vi "Teleop.vi"(10 "Match Info":T1={"Autonomous Elapsed Seconds"=0.0, "TeleOp Elapsed Seconds"=59.323, "Disabled Elapsed Seconds"=2.887, "Visited Autonomous"=FALSE, "Visited TeleOp"=TRUE, "Visited Disabled"=TRUE, "Autonomous Settings"={"Autonomous Style"=enum."Independent", "VI Refnum"=refnum}}, 11 "Call Context":T2=enum."Stop") -> ()   [LabVIEW 2018]
doc: "This VI is called for each enabled TeleOp packet received from the DS. It is typically used to read from joysticks and other inputs and update I/O or setpoints for timed control loops. It should complete and return within 20 milliseconds or risk missing DS packets."
uses:
  <vilib>/Rock Robotics/WPI/DriverStation/WPI_DriverStationDerivedRobotMode.ctl
  <vilib>/Rock Robotics/WPI/DriverStation/WPI_DriverStationMatch Info.ctl
  Typedef/XBox Axis.ctl
  Typedef/XBox Buttons.ctl
  <vilib>/Rock Robotics/WPI/ThirdParty/REV Robotics/SPARK MAX/Typedef/Spark MAX Idle Mode.ctl
  <vilib>/Rock Robotics/WPI/Solenoid/WPI_SolenoidValue.ctl
  <vilib>/Rock Robotics/WPI/Utilities/WPI_GetSetVariantRefNum.vi
  <vilib>/Rock Robotics/Network Tables/NT Write Boolean Array.vi
  <vilib>/Rock Robotics/Network Tables/NT Write Numeric Array.vi
  <vilib>/Rock Robotics/Network Tables/NT Read Number.vi
  <vilib>/Rock Robotics/Network Tables/NT Write Number.vi
  <vilib>/Rock Robotics/WPI/Solenoid/WPI_SolenoidSetEnum.vi
  Beak/Implementation/Beak Published Globals.vi
  Wrist/Implementation/Wrist Published Globals.vi
panel:
  in  "Max Acceleration":dbl=800.0
  in  "Max Velocity":dbl=400.0
  in  "Arm angle from 'Y'":dbl=86.0 format="%#_13g"
  in  "Joystick Deadband":dbl=0.07 format="%#_13g"
  in  "Throttle Sensitivity":dbl(slide)=0.7142857142857142 scale=0.0..1.0
  in  "Elevator Speed":dbl=1.5 format="%#_13g"
  in  "QuesoTurn Sensitivty":dbl=0.7
  in  "Cheesy Sensitivity":dbl(slide)=0.5864661654135338 scale=0.0..1.0
  in  "Arcade to Queso":bool=TRUE
  # "<-- This is not motor speed!"
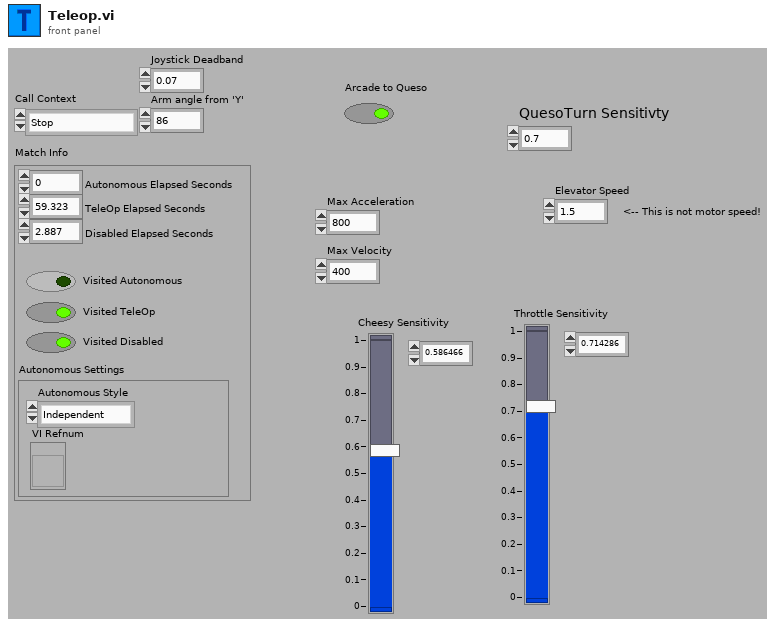
[diagram p1: front panel]
types:
  T1 = typedef "WPI_DriverStationMatch Info.ctl" = cluster{"Autonomous Elapsed Seconds":dbl, "TeleOp Elapsed Seconds":dbl, "Disabled Elapsed Seconds":dbl, "Visited Autonomous":bool, "Visited TeleOp":bool, "Visited Disabled":bool, "Autonomous Settings":cluster{"Autonomous Style":enum16{"Iterative", "Independent"}, "VI Refnum":refnum<vi>}}
  T2 = typedef "WPI_DriverStationDerivedRobotMode.ctl" = enum16{"Init", "Execute", "Stop"}
  T3 = typedef "XBox Buttons.ctl" = enum16{"A", "B", "X", "Y", "Left Bumper", "Right Bumper", "Back", "Start", "Left Joystick", "Right Joystick"}
  T4 = typedef "XBox Axis.ctl" = enum16{"Left X", "Left Y", "Left Trigger", "Right Trigger", "Right X", "Right Y"}
  T5 = typedef "WPI_JoystickDevRef.ctl" = cluster{"Device":T6}
  T6 = typedef "WPI_JoystickDeviceEnum.ctl" = enum16{"USB 0", "USB 1", "USB 2", "USB 3", "USB 4", "USB 5"}
  T7 = typedef "Spark MAX Idle Mode.ctl" = enum16{"Coast", "Brake"}
  T8 = typedef "SPARKMAX6Motor.ctl" = cluster{"FrontLeftMaster":T9, "FrontLeftSlave1":T9, "FrontLeftSlave2":T9, "FrontRightMaster":T9, "FrontRightSlave1":T9, "FrontRightSlave2":T9}
  T9 = typedef "WPI_MotorControlDeviceRef.ctl" = cluster{"DeviceStatus":errorcluster, "Type":T10, "PWM":cluster{"PWM Channel":T11, "DeadBand":T12}, "CAN":cluster{"Device Number":u8, "SetOutput VI Ref":variant, "GetOutput VI Ref":variant, "Enable VI Ref":variant, "Disable VI Ref":variant, "Data":variant}, "Invert":bool, "DIO PWM":cluster{"PWM \"Enable\" Channel":T11, "DIOChannel":T13, "PWM Rate":dbl}}
  T10 = typedef "WPI_MotorControlType.ctl" = enum16{"PWM", "CAN", "DIO PWM"}
  T11 = typedef "FPGA_DIOPWMChannel.ctl" = enum8{"PWM 0", "PWM 1", "PWM 2", "PWM 3", "PWM 4", "PWM 5", "PWM 6", "PWM 7", "PWM 8", "PWM 9", "PWM MXP 0", "PWM MXP 1", "PWM MXP 2", "PWM MXP 3", "PWM MXP 4", "PWM MXP 5", "PWM MXP 6", "PWM MXP 7", "PWM MXP 8", "PWM MXP 9", "Invalid"}
  T12 = typedef "WPI_PWMDeadband.ctl" = cluster{"Name":string, "maxPositivePwm":i32, "minPositivePwm":i32, "centerPwm":i32, "maxNegativePwm":i32, "minNegativePwm":i32, "angularRange":u16}
  T13 = typedef "FPGA_DIOChannel.ctl" = enum8{"DIO 0", "DIO 1", "DIO 2", "DIO 3", "DIO 4", "DIO 5", "DIO 6", "DIO 7", "DIO 8", "DIO 9", "DIO MXP 0", "DIO MXP 1", "DIO MXP 2", "DIO MXP 3", "DIO MXP 4", "DIO MXP 5", "DIO MXP 6", "DIO MXP 7", "DIO MXP 8", "DIO MXP 9", "DIO MXP 10", "DIO MXP 11", "DIO MXP 12", "DIO MXP 13", "DIO MXP 14", "DIO MXP 15", "SPI Port CS1", "SPI Port CS2", "SPI Port CS3", "SPI Port MISO", "SPI Port MOSI", "Invalid"}
  T14 = typedef "WPI_SolenoidValue.ctl" = enum16{"Off", "On", "Forward", "Reverse"}
  T15 = typedef "WPI_SolenoidDevRef.ctl" = cluster{"DevStatus":errorcluster, "Pneumatics Control Module":u8, "Forward Solenoid Channel":T16, "Reverse Solenoid Channel":T16}
  T16 = typedef "WPI_SolenoidChannel.ctl" = enum8{"Solenoid 0", "Solenoid 1", "Solenoid 2", "Solenoid 3", "Solenoid 4", "Solenoid 5", "Solenoid 6", "Solenoid 7", "Invalid"}
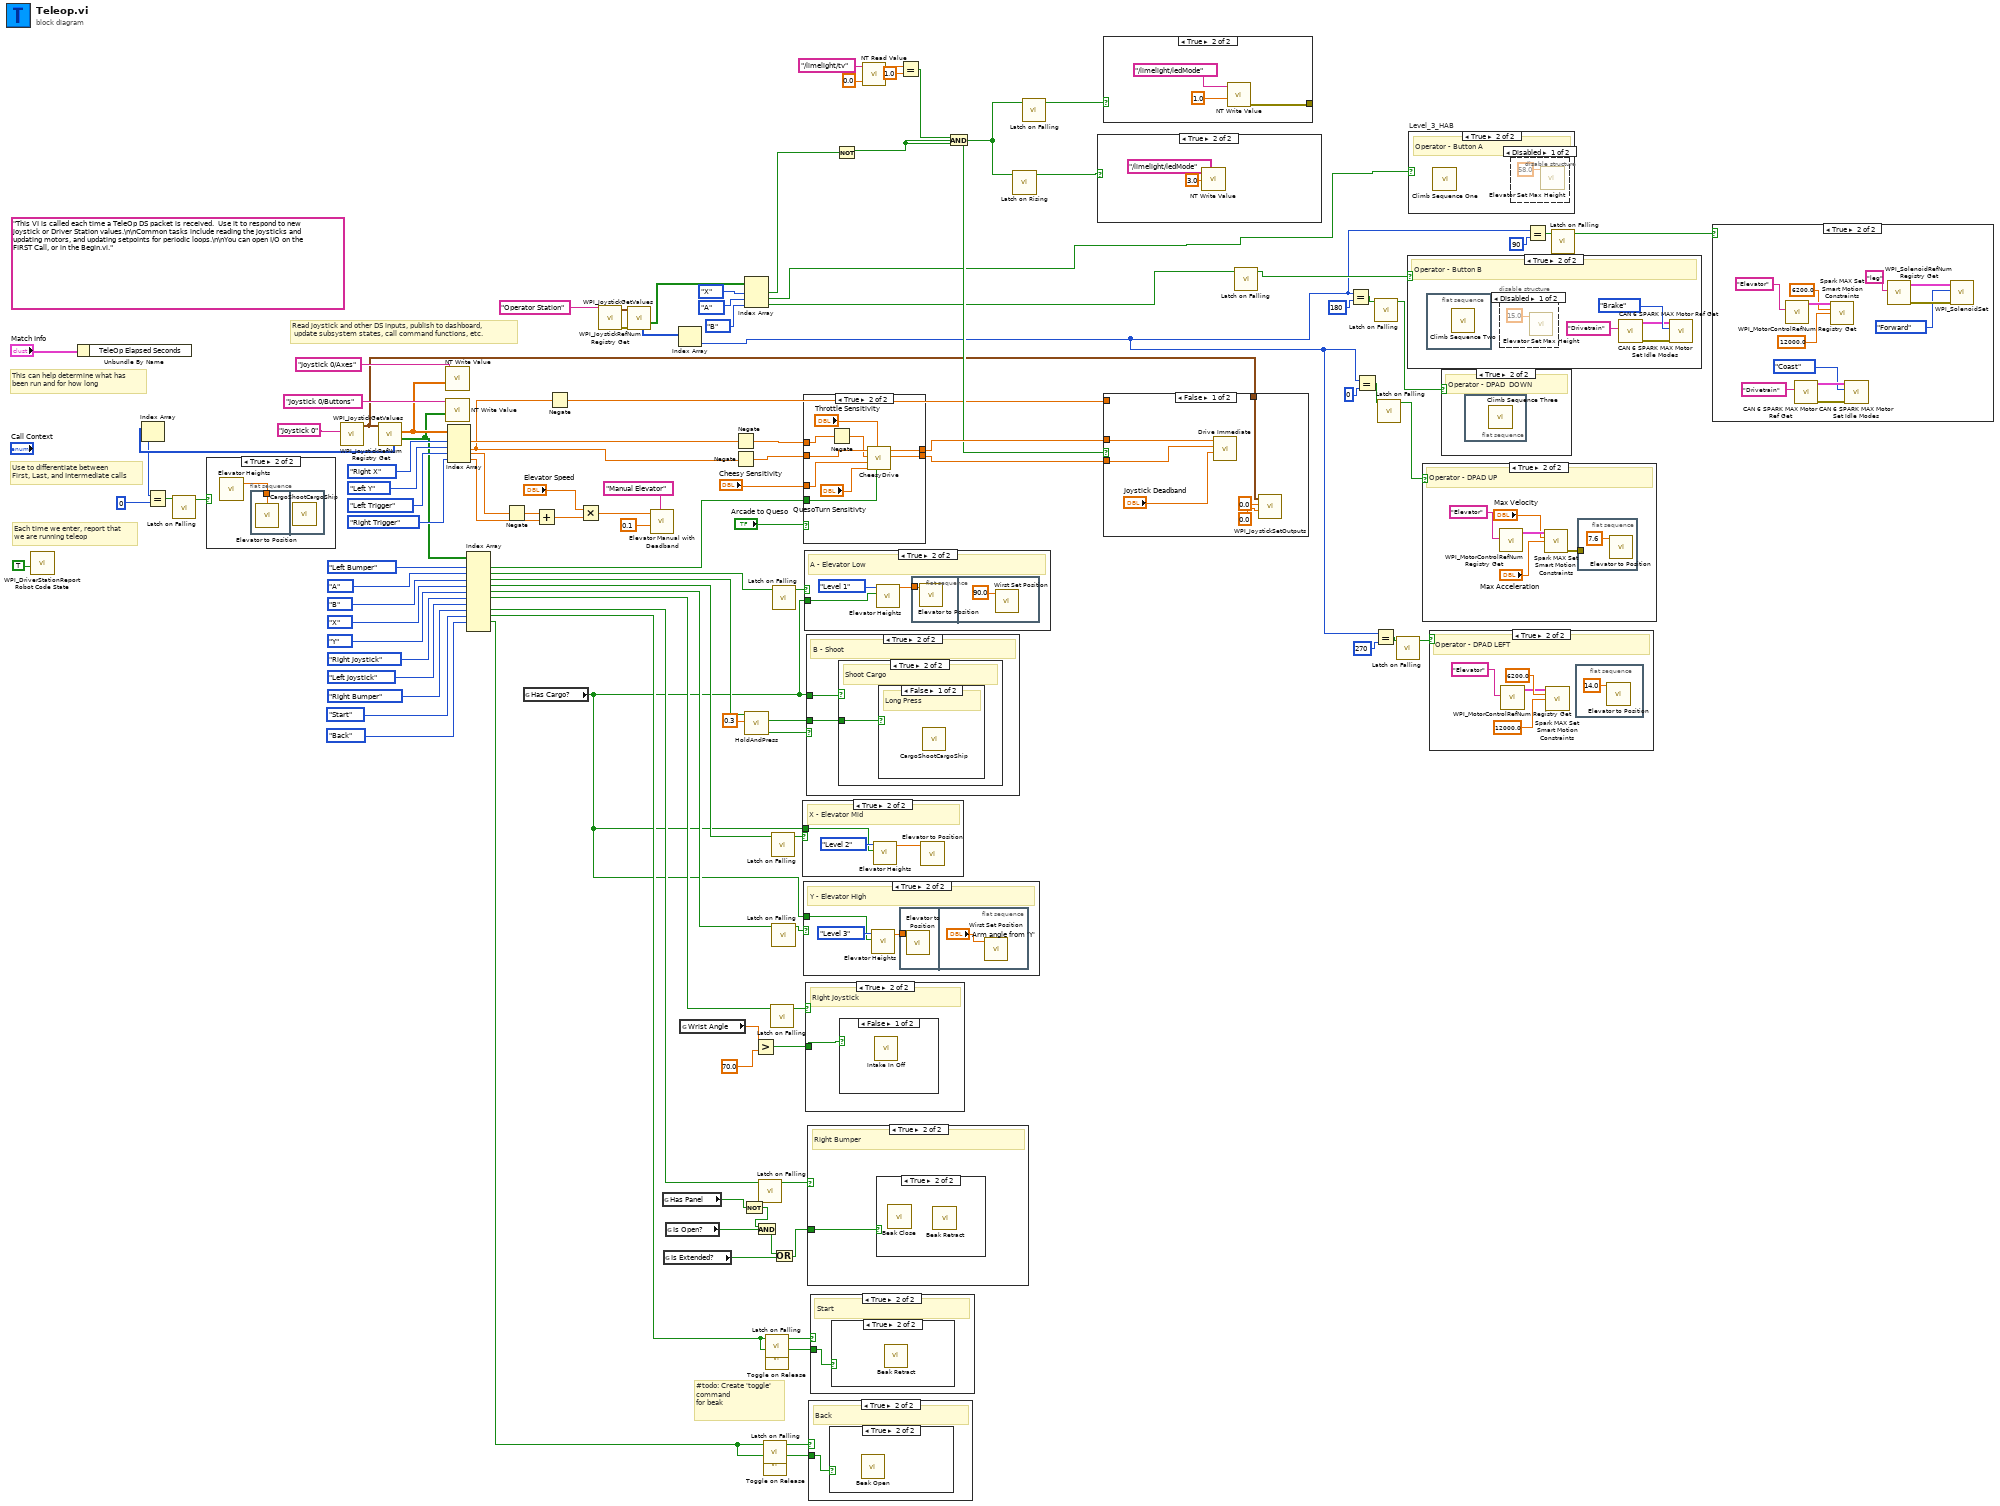
[diagram p0: block diagram]
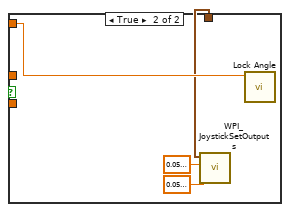
[diagram p13: hidden frame]
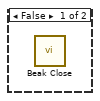
[diagram p16: hidden frame]
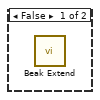
[diagram p18: hidden frame]
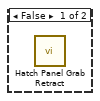
[diagram p20: hidden frame]
diagram:
  (unwired) "This VI is called each time a TeleOp DS packet is received.  Use it to respond to new joystick or Driver Station values.\n\nCommon tasks include reading the joysticks and updating motors, and updating setpoints for periodic loops.\n\nYou can open I/O on the FIRST Call, or in the Begin.vi."
  # "#todo: Create 'toggle' command\nfor beak"
  # "Read joystick and other DS inputs, publish to dashboard,\n update subsystem states, call command functions, etc."
  # "Each time we enter, report that\nwe are running teleop"
  # "Use to differentiate between\nFirst, Last, and Intermediate calls"
  # "This can help determine what has\nbeen run and for how long"
  n1 = call <vilib>:"WPI_DriverStationReport Robot Code State.vi"("TeleOp"=TRUE ("Autonomous")) -> ()  [unwired: 10 in, 1 out]
  n2 = Unbundle By Name("Match Info") -> ()  [unwired: 1 out]
  n3 = call <vilib>:"WPI_JoystickRefNum Registry Get.vi"("refnum name"="Joystick 0") -> ("JoystickDevRef"=w30:T5)  [unwired: 1 in, 9 out]
  n4 = call <vilib>:"WPI_JoystickGetValues.vi"("JoystickDevRef"=w30) -> ("Buttons"=w84:bool[], "Axes"=w105:dbl[], "POVs"=w19:i16[])  [unwired: 6 in, 2 out]
  n5 = Index Array(array=w19) -> (element=w18:i16)  [unwired: 1 in]
  n6 = Equal?(x=w18, y=0) -> (x = y?=w17:bool)
  n7 = call "Latch on Falling.vi"("Boolean in"=w17) -> ("Boolean out"=w16:bool)  [unwired: 4 in]
  n8 = case shown="True" w16 {
    frame False {
    }
    frame True {
      n9 = call "Elevator Heights.vi"() -> ("Cargo Ship Height"=w110:dbl)  [unwired: 10 in, 1 out]
      n10 = flat-sequence {
        tunnel: w110 -> [w111]
        frame #0 {
          n11 = call "Elevator to Position.vi"("Elevator Height"=w111) -> ()  [unwired: 10 in, 1 out]
        }
        frame #1 {
          n12 = call "CargoShootCargoShip.vi"() -> ()  [unwired: 11 in, 1 out]
        }
      }
    }
  }
  n13 = call-poly <vilib>:"NT Write Value.vi"("Numeric Array"=w105, "Name"="Joystick 0/Axes") -> ()  [unwired: 9 in, 1 out]
  n14 = call-poly <vilib>:"NT Write Value.vi"("Boolean Array"=w84, "Name"="Joystick 0/Buttons") -> ()  [unwired: 9 in, 1 out]
  n15 = Index Array(array=w105, index #1=XBox_Axis."Right X" ("Enum"), index #2=XBox_Axis."Left Y" ("Enum"), index #3=XBox_Axis."Left Trigger" ("Enum"), index #4=XBox_Axis."Right Trigger" ("Enum")) -> (element #1=w101:dbl, element #2=w29:dbl, element #3=w89:dbl, element #4=w88:dbl)
  n16 = Index Array(array=w84, index #1=XBox_Buttons."Left Bumper" ("Enum"), index #2=XBox_Buttons."A" ("Enum"), index #3=XBox_Buttons."B" ("Enum"), index #4=XBox_Buttons."X" ("Enum"), index #5=XBox_Buttons."Y" ("Enum"), index #6=XBox_Buttons."Right Joystick" ("Enum"), index #7=XBox_Buttons."Left Joystick" ("Enum"), index #8=XBox_Buttons."Right Bumper" ("Enum"), index #9=XBox_Buttons."Start" ("Enum"), index #10=XBox_Buttons."Back" ("Enum")) -> (element #1=w77:bool, element #2=w76:bool, element #3=w59:bool, element #4=w73:bool, element #5=w72:bool, element #6=w60:bool, element #8=w68:bool, element #9=w64:bool, element #10=w61:bool)  [unwired: 1 in, 2 out]
  n17 = Negate(x=w89) -> (-x=w86:dbl)
  n18 = global read "Wrist Published Globals.vi" "Has Cargo?"() -> (w49:bool)
  n19 = Add(x=w86, y=w88) -> (x+y=w87:dbl)
  n20 = Negate(x=w29) -> (-x=w28:dbl)
  n21 = Multiply(x="Elevator Speed", y=w87) -> (x*y=w80:dbl)
  n22 = call <vilib>:"WPI_JoystickRefNum Registry Get.vi"("refnum name"="Operator Station") -> ("error out"=w44:errorcluster, "JoystickDevRef"=w43:T5)  [unwired: 9 in]
  n23 = call <vilib>:"WPI_JoystickGetValues.vi"("error in (no error)"=w44, "JoystickDevRef"=w43) -> ("Buttons"=w39:bool[], "POVs"=w23:i16[])  [unwired: 5 in, 3 out]
  n24 = call "Elevator Manual with Deadband.vi"("Description"="Manual Elevator", "Deadband Value"=0.1, "Setpoint"=w80) -> ()  [unwired: 8 in, 1 out]
  n25 = global read "Beak Published Globals.vi" "Has Panel"() -> (w53:bool)
  n26 = global read "Beak Published Globals.vi" "Is Extended?"() -> (w54:bool)
  n27 = global read "Beak Published Globals.vi" "Is Open?"() -> (w50:bool)
  n28 = Index Array(array=w23) -> (element=w1:i16)  [unwired: 1 in]
  n29 = global read "Wrist Published Globals.vi" "Wrist Angle"() -> (w47:dbl)
  n30 = Negate(x=w101) -> (-x=w99:dbl)
  n31 = Negate(x=w29) -> (-x=w100:dbl)
  n32 = Not(x=w53) -> (.not. x?=w52:bool)
  n33 = Index Array(array=w39, index #1=XBox_Buttons."X" ("Enum"), index #2=XBox_Buttons."A" ("Enum"), index #3=XBox_Buttons."B" ("Enum")) -> (element #1=w37:bool, element #2=w14:bool, element #3=w21:bool)
  n34 = call "HoldAndPress.vi"("Holdtime"=0.3, "Input"=w59) -> ("Press?"=w57:bool, "Quick Press"=w56:bool)  [unwired: 4 in, 4 out]
  n35 = Greater?(x=w47, y=70.0) -> (0:w45:bool)
  n36 = And(x=w52, y=w50) -> (x .and. y?=w51:bool)
  n37 = call "Latch on Falling.vi"("Boolean in"=w68) -> ("Boolean out"=w70:bool)  [unwired: 4 in]
  n38 = call "Latch on Falling.vi"("Boolean in"=w61) -> ("Boolean out"=w62:bool)  [unwired: 4 in]
  n39 = call "Toggle on Release.vi"("Boolean"=w61) -> ("toggle on release"=w63:bool)  [unwired: 10 in]
  n40 = call "Latch on Falling.vi"("Boolean in"=w64) -> ("Boolean out"=w69:bool)  [unwired: 4 in]
  n41 = call "Toggle on Release.vi"("Boolean"=w64) -> ("toggle on release"=w67:bool)  [unwired: 10 in]
  n42 = call "Latch on Falling.vi"("Boolean in"=w60) -> ("Boolean out"=w71:bool)  [unwired: 4 in]
  n43 = call "Latch on Falling.vi"("Boolean in"=w73) -> ("Boolean out"=w74:bool)  [unwired: 4 in]
  n44 = call "Latch on Falling.vi"("Boolean in"=w72) -> ("Boolean out"=w48:bool)  [unwired: 4 in]
  n45 = call "Latch on Falling.vi"("Boolean in"=w76) -> ("Boolean out"=w75:bool)  [unwired: 4 in]
  n46 = Or(x=w51, y=w54) -> (x .or. y?=w55:bool)
  n47 = case shown="True" w74 {
    tunnel: w49 -> [_ w112]
    frame False {
    }
    frame True {
      # "X - Elevator Mid"
      n48 = call "Elevator Heights.vi"("With Cargo?"=w112, "Level"=enum16{"Level 1", "Level 2", "Level 3"}."Level 2") -> ("Height"=w114:dbl)  [unwired: 8 in, 1 out]
      n49 = call "Elevator to Position.vi"("Elevator Height"=w114) -> ()  [unwired: 10 in, 1 out]
    }
  }
  n50 = case shown="True" "Arcade to Queso" {
    tunnel: w100 -> [w118 w125]
    tunnel: w99 -> [w119 w124]
    tunnel: [w117 w128] -> w41
    tunnel: [w116 w127] -> w40
    tunnel: w77 -> [_ w126]
    tunnel: "Cheesy Sensitivity" -> [_ w122]
    frame False {
      n51 = call <vilib>:"WPI_JoystickArcadeMapping.vi"("Square Inputs"=FALSE, "Y axis value"=w118, "X axis value"=w119) -> ("Right Motor Value"=w117:dbl, "Left Motor Value"=w116:dbl)  [unwired: 7 in]
    }
    frame True {
      n52 = Negate(x=w124) -> (-x=w123:dbl)
      n53 = call "CheesyDrive.vi"("Quickturn"=w126, "Throttle Sensitivity"="Throttle Sensitivity", "QuickTurn Sensitivty"="QuesoTurn Sensitivty", "Queso Arc Sensitivty"=w122, "Wheel"=w123, "Throttle"=w125) -> ("Right PWM"=w128:dbl, "Left PWM"=w127:dbl)  [unwired: 4 in]
    }
  }
  n54 = case shown="True" w48 {
    tunnel: w49 -> [_ w129]
    frame False {
    }
    frame True {
      # "Y - Elevator High"
      n55 = call "Elevator Heights.vi"("With Cargo?"=w129, "Level"=enum16{"Level 1", "Level 2", "Level 3"}."Level 3") -> ("Height"=w131:dbl)  [unwired: 8 in, 1 out]
      n56 = flat-sequence {
        tunnel: w131 -> [w132]
        frame #0 {
          n57 = call "Elevator to Position.vi"("Elevator Height"=w132) -> ()  [unwired: 10 in, 1 out]
        }
        frame #1 {
          n58 = call "Wirst Set Position.vi"("Setpoint (Degrees)"="Arm angle from 'Y'") -> ()  [unwired: 10 in, 1 out]
        }
      }
    }
  }
  n59 = case shown="True" w75 {
    tunnel: w49 -> [_ w134]
    frame False {
    }
    frame True {
      # "A - Elevator Low"
      n60 = call "Elevator Heights.vi"("With Cargo?"=w134, "Level"=enum16{"Level 1", "Level 2", "Level 3"}."Level 1") -> ("Height"=w136:dbl)  [unwired: 8 in, 1 out]
      n61 = flat-sequence {
        tunnel: w136 -> [w137]
        frame #0 {
          n62 = call "Elevator to Position.vi"("Elevator Height"=w137) -> ()  [unwired: 10 in, 1 out]
        }
        frame #1 {
          n63 = call "Wirst Set Position.vi"("Setpoint (Degrees)"=90.0) -> ()  [unwired: 10 in, 1 out]
        }
      }
    }
  }
  n64 = case shown="True" w71 {
    tunnel: w45 -> [_ w139]
    frame False {
    }
    frame True {
      # "Right Joystick"
      n65 = case shown="False" w139 {
        frame False {
          n66 = call "Intake In Off.vi"() -> ()  [unwired: 11 in, 1 out]
        }
        frame True {
          n67 = call "Intake Deploy On.vi"() -> ()  [unwired: 11 in, 1 out]
        }
      }
    }
  }
  n68 = case shown="True" w57 {
    tunnel: w56 -> [_ w141]
    tunnel: w49 -> [_ w140]
    frame False {
    }
    frame True {
      # "B - Shoot"
      n69 = case shown="True" w140 {
        tunnel: w141 -> [w142 w143]
        frame False {
          # "Score Hatch Panel"
          n70 = case shown="False" w142 {
            frame False {
              # "Long Press"
              n71 = call "Hatch Panel Score.vi"() -> ()  [unwired: 11 in, 1 out]
            }
            frame True {
              # "Quick Press?"
              n72 = call "Beak Close.vi"() -> ()  [unwired: 11 in, 1 out]
            }
          }
        }
        frame True {
          # "Shoot Cargo"
          n73 = case shown="False" w143 {
            frame False {
              # "Long Press"
              n74 = call "CargoShootCargoShip.vi"() -> ()  [unwired: 11 in, 1 out]
            }
            frame True {
              # "Quick Press"
              n75 = call "Cargo Shoot.vi"() -> ()  [unwired: 11 in, 1 out]
            }
          }
        }
      }
    }
  }
  n76 = case shown="True" w70 {
    tunnel: w55 -> [_ w144]
    frame False {
    }
    frame True {
      # "Right Bumper"
      n77 = case shown="True" w144 {
        frame False {
          n78 = call "Hatch Panel Grab Retract.vi"() -> ()  [unwired: 11 in, 1 out]
        }
        frame True {
          n79 = call "Beak Close.vi"() -> ()  [unwired: 11 in, 1 out]
          n80 = call "Beak Retract.vi"() -> ()  [unwired: 11 in, 1 out]
        }
      }
    }
  }
  n81 = case shown="True" w62 {
    tunnel: w63 -> [_ w145]
    frame False {
    }
    frame True {
      # "Back"
      n82 = case shown="True" w145 {
        frame False {
          n83 = call "Beak Close.vi"() -> ()  [unwired: 11 in, 1 out]
        }
        frame True {
          n84 = call "Beak Open.vi"() -> ()  [unwired: 11 in, 1 out]
        }
      }
    }
  }
  n85 = case shown="True" w69 {
    tunnel: w67 -> [_ w146]
    frame False {
    }
    frame True {
      # "Start"
      n86 = case shown="True" w146 {
        frame False {
          n87 = call "Beak Extend.vi"() -> ()  [unwired: 11 in, 1 out]
        }
        frame True {
          n88 = call "Beak Retract.vi"() -> ()  [unwired: 11 in, 1 out]
        }
      }
    }
  }
  n89 = Not(x=w37) -> (.not. x?=w26:bool)
  n90 = call-poly <vilib>:"NT Read Value.vi"("Default Value"=0.0, "Name"="/limelight/tv") -> ("Numeric"=w34:dbl)  [unwired: 8 in, 1 out]
  n91 = Equal?(x=w34, y=1.0) -> (x = y?=w32:bool)
  n92 = And(x=w32, y=w26) -> (x .and. y?=w31:bool)
  n93 = call "Latch on Rising.vi"("Boolean in"=w26) -> ("Boolean out"=w27:bool)  [unwired: 4 in]
  n94 = call "Latch on Falling.vi"("Boolean in"=w26) -> ("Boolean out"=w25:bool)  [unwired: 4 in]
  n95 = case shown="True" w27 {
    frame False {
    }
    frame True {
      n96 = call-poly <vilib>:"NT Write Value.vi"("Numeric"=3.0, "Name"="/limelight/ledMode") -> ()  [unwired: 9 in, 1 out]
    }
  }
  n97 = case shown="True" w25 {
    tunnel: [_ w149] -> _
    frame False {
    }
    frame True {
      n98 = call-poly <vilib>:"NT Write Value.vi"("Numeric"=1.0, "Name"="/limelight/ledMode") -> ("error out"=w149:errorcluster)  [unwired: 9 in]
    }
  }
  n99 = case shown="False" w31 {
    tunnel: w41 -> [w156 _]
    tunnel: w40 -> [w155 _]
    tunnel: w28 -> [_ w161]
    tunnel: w30 -> [w152 w158]
    frame False {
      n100 = call "Drive Immediate.vi"("Deadband Value"="Joystick Deadband", "Right Setpoint"=w156, "Left Setpoint"=w155) -> ()  [unwired: 8 in, 1 out]
      n101 = call <vilib>:"WPI_JoystickSetOutputs.vi"("Right Rumble"=sgl 0.0, "Left Rumble"=sgl 0.0, "JoystickDevRef"=w152) -> ()  [unwired: 7 in, 2 out]
    }
    frame True {
      n102 = call <vilib>:"WPI_JoystickSetOutputs.vi"("Right Rumble"=sgl 0.05, "Left Rumble"=sgl 0.05, "JoystickDevRef"=w158) -> ()  [unwired: 7 in, 2 out]
      n103 = call "Lock Angle.vi"("Setpoint"=w161) -> ()  [unwired: 11 in]
    }
  }
  n104 = call "Latch on Falling.vi"("Boolean in"=w21) -> ("Boolean out"=w13:bool)  [unwired: 4 in]
  n105 = Equal?(x=w1, y=i16 180 ("element")) -> (x = y?=w11:bool)
  n106 = Equal?(x=w1, y=i16 0 ("element")) -> (x = y?=w10:bool)
  n107 = Equal?(x=w1, y=i16 270 ("element")) -> (x = y?=w3:bool)
  n108 = call "Latch on Falling.vi"("Boolean in"=w11) -> ("Boolean out"=w15:bool)  [unwired: 4 in]
  n109 = call "Latch on Falling.vi"("Boolean in"=w10) -> ("Boolean out"=w8:bool)  [unwired: 4 in]
  n110 = call "Latch on Falling.vi"("Boolean in"=w3) -> ("Boolean out"=w2:bool)  [unwired: 4 in]
  n111 = case shown="True" w13 {
    frame False {
    }
    frame True {
      # "Operator - Button B"
      n112 = flat-sequence {
        frame #0 {
          n113 = call "Climb Sequence Two.vi"() -> ()  [unwired: 11 in, 1 out]
        }
      }
      n114 = disable-structure shown="Disabled" {
        frame Disabled {
          n115 = call "Elevator Set Max Height.vi"("Setpoint"=15.0) -> ()  [unwired: 10 in, 1 out]
        }
        frame Enabled {
        }
      }
      n116 = call "CAN 6 SPARK MAX Motor Ref Get.vi"("refnum name"="Drivetrain") -> ("error out"=w162:errorcluster, "TalonSRX6MotorRef out"=w163:T8)  [unwired: 9 in]
      n117 = call "CAN 6 SPARK MAX Motor Set Idle Modes.vi"("error in (no error)"=w162, "Idle Mode"=Spark_MAX_Idle_Mode."Brake", "SPARK MAX ref in"=w163) -> ()  [unwired: 7 in, 2 out]
    }
  }
  n118 = case "Level_3_HAB" shown="True" w14 {
    frame False {
    }
    frame True {
      # "Operator - Button A"
      n119 = call "Climb Sequence One.vi"() -> ()  [unwired: 11 in, 1 out]
      n120 = disable-structure shown="Disabled" {
        frame Disabled {
          n121 = call "Elevator Set Max Height.vi"("Setpoint"=58.0) -> ()  [unwired: 10 in, 1 out]
        }
        frame Enabled {
        }
      }
    }
  }
  n122 = case shown="True" w8 {
    frame False {
    }
    frame True {
      # "Operator - DPAD UP"
      n123 = call <vilib>:"WPI_MotorControlRefNum Registry Get.vi"("refnum name"="Elevator") -> ("MotorControlDevRef"=w172:T9)  [unwired: 9 in, 1 out]
      n124 = call <vilib>:"Spark MAX Set Smart Motion Constraints.vi"("MotorControlDeviceRef"=w172, "Max Velocity"="Max Velocity", "Max Acceleration"="Max Acceleration") -> ("error out"=w168:errorcluster)  [unwired: 11 in, 1 out]
      n125 = flat-sequence {
        tunnel: w168 -> [_]
        frame #0 {
          n126 = call "Elevator to Position.vi"("Elevator Height"=7.6) -> ()  [unwired: 10 in, 1 out]
        }
      }
    }
  }
  n127 = case shown="True" w2 {
    frame False {
    }
    frame True {
      # "Operator - DPAD LEFT"
      n128 = call <vilib>:"WPI_MotorControlRefNum Registry Get.vi"("refnum name"="Elevator") -> ("MotorControlDevRef"=w175:T9)  [unwired: 9 in, 1 out]
      n129 = call <vilib>:"Spark MAX Set Smart Motion Constraints.vi"("MotorControlDeviceRef"=w175, "Max Velocity"=6200.0, "Max Acceleration"=12000.0) -> ()  [unwired: 11 in, 2 out]
      n130 = flat-sequence {
        frame #0 {
          n131 = call "Elevator to Position.vi"("Elevator Height"=14.0) -> ()  [unwired: 10 in, 1 out]
        }
      }
    }
  }
  n132 = case shown="True" w15 {
    frame False {
    }
    frame True {
      # "Operator - DPAD  DOWN"
      n133 = flat-sequence {
        frame #0 {
          n134 = call "Climb Sequence Three.vi"() -> ()  [unwired: 11 in, 1 out]
        }
      }
    }
  }
  n135 = Equal?(x=w1, y=i16 90 ("element")) -> (x = y?=w6:bool)
  n136 = call "Latch on Falling.vi"("Boolean in"=w6) -> ("Boolean out"=w5:bool)  [unwired: 4 in]
  n137 = case shown="True" w5 {
    frame False {
    }
    frame True {
      n138 = call <vilib>:"WPI_MotorControlRefNum Registry Get.vi"("refnum name"="Elevator") -> ("MotorControlDevRef"=w189:T9)  [unwired: 9 in, 1 out]
      n139 = call "CAN 6 SPARK MAX Motor Ref Get.vi"("refnum name"="Drivetrain") -> ("error out"=w186:errorcluster, "TalonSRX6MotorRef out"=w185:T8)  [unwired: 9 in]
      n140 = call <vilib>:"Spark MAX Set Smart Motion Constraints.vi"("MotorControlDeviceRef"=w189, "Max Velocity"=6200.0, "Max Acceleration"=12000.0) -> ()  [unwired: 11 in, 2 out]
      n141 = call "CAN 6 SPARK MAX Motor Set Idle Modes.vi"("error in (no error)"=w186, "Idle Mode"=Spark_MAX_Idle_Mode."Coast", "SPARK MAX ref in"=w185) -> ()  [unwired: 7 in, 2 out]
      n142 = call <vilib>:"WPI_SolenoidRefNum Registry Get.vi"("refnum name"="leg") -> ("error out"=w180:errorcluster, "SolenoidDevRef"=w182:T15)  [unwired: 9 in]
      n143 = call-poly <vilib>:"WPI_SolenoidSet.vi"("error in (no error)"=w180, "Value"=WPI_SolenoidValue."Forward", "SolenoidDevRef"=w182) -> ()  [unwired: 7 in, 2 out]
    }
  }
